vi "filter.test.vi"(9 "reset":bool, 10 "debug":bool) -> ()   [LabVIEW 2022 SP3]
uses:
  <vilib>/Platform/TimedLoop/XDataNode/timing_clust.ctl
  <vilib>/Platform/TimedLoop/XDataNode/nitl_modes.ctl
  <vilib>/Platform/TimedLoop/XDataNode/wakeup.ctl
  ticker.slot.ctl
  arty/orderbook/orderbook.command.ctl
  arty/orderbook/orderbook.command.type.ctl
  <vilib>/rvi/DataTransferAndStorage/Container/Common/niFpgaContainerGetUniqueNameForEmu.vi
  <vilib>/rvi/DataTransferAndStorage/Container/Common/niFpgaContainerSetEmuInfo.vi
  <vilib>/rvi/eio/common/nirviEmuReportErrorAndStop.vi
  <vilib>/rvi/Emulation/niFpgaSctlEmulationGetInTimedLoop.vi
  <vilib>/rvi/Emulation/niFpgaEmulationReportErrorSimple.vi
  <vilib>/rvi/Emulation/niFpgaGetClockAttributes.vi
  <vilib>/rvi/Emulation/niFpgaCriticalErrorInLSC.vi
  <vilib>/rvi/DataTransferAndStorage/Container/Common/niFpgaContainerExecOnDevCompGetState.vi
  <vilib>/rvi/Emulation/niFpgaEmulationIsFPGAContextNoSignature.vi
  <vilib>/rvi/errors/niFpgaSetErrorForExecOnDevCompSimple.vi
  <vilib>/rvi/FIFO/Fifo_Resource/nirvififoEmulationSetSize.vi
  <vilib>/rvi/FIFO/Fifo_Resource/nirviFifoEmulationQueueMgr.vi
  <instcachedir>/0/nirviFifoEmulationQueueMgr_E5CAEC123FF24DC58D834DCA3CDAA9B5.lvgen/nirviFifoEmulationQueueMgr_E5CAEC123FF24DC58D834DCA3CDAA9B5_012.vi
  <vilib>/rvi/FIFO/Fifo_Resource/nirvififoEmulationDetermineInputValidOut.vi
  <vilib>/rvi/FIFO/Fifo_Resource/nirvififoEmulationCreateLock.vi
  <vilib>/rvi/Emulation/niFpgaProcessEmulError.vi
  <vilib>/rvi/FIFO/Fifo_Resource/nirvififoEmulationObtainLock.vi
  <vilib>/rvi/FIFO/Fifo_Resource/nirvififoEmulationReleaseLock.vi
  <vilib>/rvi/occurrence/nirviWaitOnOccurrenceBase.vi
  <vilib>/rvi/errors/nirviReportUnexpectedCaseInternalError.vi
  <vilib>/rvi/errors/nirviReportUnexpectedCaseInternalError (U32).vi
  <vilib>/Utility/error.llb/Clear Errors.vi
  <vilib>/rvi/interface/RandomDataEmulation/niFpgaRandomDataHandleErrors.vi
  <instcachedir>/0/nirviFifoEmulationQueueMgr_E5CAEC123FF24DC58D834DCA3CDAA9B5.lvgen/nirviFifoEmulationQueueMgr_E5CAEC123FF24DC58D834DCA3CDAA9B5_011.vi
  <vilib>/rvi/interface/RandomDataEmulation/nirviRandomDataMultiElementFPGAFIFO.vi
  <instcachedir>/0/nirviRandomDataMultiElementFPGAFIFO_3E9965BA1FAD4E7B8DABA31768A09B1F.lvgen/nirviRandomDataMultiElementFPGAFIFO_3E9965BA1FAD4E7B8DABA31768A09B1F_001.vi
  <instcachedir>/0/nirviFifoEmulationQueueMgr_E5CAEC123FF24DC58D834DCA3CDAA9B5.lvgen/nirviFifoEmulationQueueMgr_E5CAEC123FF24DC58D834DCA3CDAA9B5_017.vi
  <vilib>/Platform/TimedLoop/XDataNode/XDataNode.xnode
  <vilib>/rvi/LocalResourceManager/LocalResourceManager.xnode
  <vilib>/rvi/DataTransferAndStorage/Container/XNode/niFpgaContainer.xnode
  <vilib>/rvi/FIFO/Fifo_Resource/niFpgaFifoEmulationRefIn.vi
  <vilib>/rvi/interface/RandomDataEmulation/nirviRandomDataFpgaReadWriteTemplate.vi
  <vilib>/rvi/FIFO/Fifo_Resource/nirvififoEmulationRead.vi
  <vilib>/rvi/interface/RandomDataEmulation/nirviRandomDataFpgaMultiElementTemplate.vi
  <vilib>/rvi/FIFO/Fifo_Resource/nirvififoEmulationWrite.vi
  <vilib>/Platform/TimedLoop/XDataNode/XDNodeRunTimeDep.lvlib
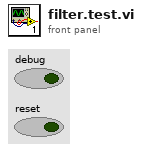
[diagram p1: front panel]
types:
  T1 = typedef "XDNodeRunTimeDep.lvlib/timing_clust.ctl" = cluster{"Expected End [f-1]":u64, "Actual End [f-1]":u64, "Finished Late? [f-1]":bool, "Expected End [i-1]":u64, "Actual End [i-1]":u64, "Finished Late? [i-1]":bool, "Expected Start [i]":u64, "Actual Start [i]":u64, "Expected Start [f]":u64, "Actual Start [f]":u64, "Source Name":string, "Structure Name":string, "Period":i64, "Deadline":i64, "Offset":i64, "Start":i64, "Priority":i32, "Timeout":i32, "Mode":T2, "Wakeup Reason":T3, "Error":errorcluster, "Source Type":string, "Secondary Source Type":string, "Global End Time":u64, "Global Start Time":u64, "Frame Duration":u64, "Iteration Duration":u64, "Assigned CPU":i32, "I/O Scan Engine Mode":u32}
  T2 = typedef "XDNodeRunTimeDep.lvlib/nitl_modes.ctl" = enum32{"No Change", "Process missed periods, maintain original phase", "Discard missed periods, maintain original phase", "Process missed periods, ignore original phase", "Discard missed periods, ignore original phase"}
  T3 = typedef "XDNodeRunTimeDep.lvlib/wakeup.ctl" = enum32{"Normal", "Aborted", "Asynchronous wakeup", "Timing source error", "Timed loop error", "Timeout"}
  T4 = typedef "orderbook.command.ctl" = cluster{"OrderBook Command.Type":T5, "Side (U8)":u8, "Order Id (U64)":u64, "Quantity (U32)":u32, "Symbol (U64)":u64, "Price (U64)":u64, "Executed Quantity (U32)":u32, "Canceled Quantity (U32)":u32, "Remaining Quantity (U32)":u32, "Seconds (U64)":u64, "Nanoseconds (U64)":u64}
  T5 = typedef "orderbook.command.type.ctl" = enum16{"Time", "AddOrder", "OrderExecuted", "OrderExecutedAtPrice", "ReduceSize", "ModifyOrder", "DeleteOrder", "Get.All.Orders", "Get.Top"}
  T6 = typedef "ticker.slot.ctl" = cluster{"Symbol":u64}
  T7 = cluster{"OrderBook Command.Type":enum16{"Time", "AddOrder", "OrderExecuted", "OrderExecutedAtPrice", "ReduceSize", "ModifyOrder", "DeleteOrder", "Get.All.Orders", "Get.Top"}, "Side (U8)":u8, "Order Id (U64)":u64, "Quantity (U32)":u32, "Symbol (U64)":u64, "Price (U64)":u64, "Executed Quantity (U32)":u32, "Canceled Quantity (U32)":u32, "Remaining Quantity (U32)":u32, "Seconds (U64)":u64, "Nanoseconds (U64)":u64}
  T8 = enum16{"Time", "AddOrder", "OrderExecuted", "OrderExecutedAtPrice", "ReduceSize", "ModifyOrder", "DeleteOrder", "Get.All.Orders", "Get.Top"}
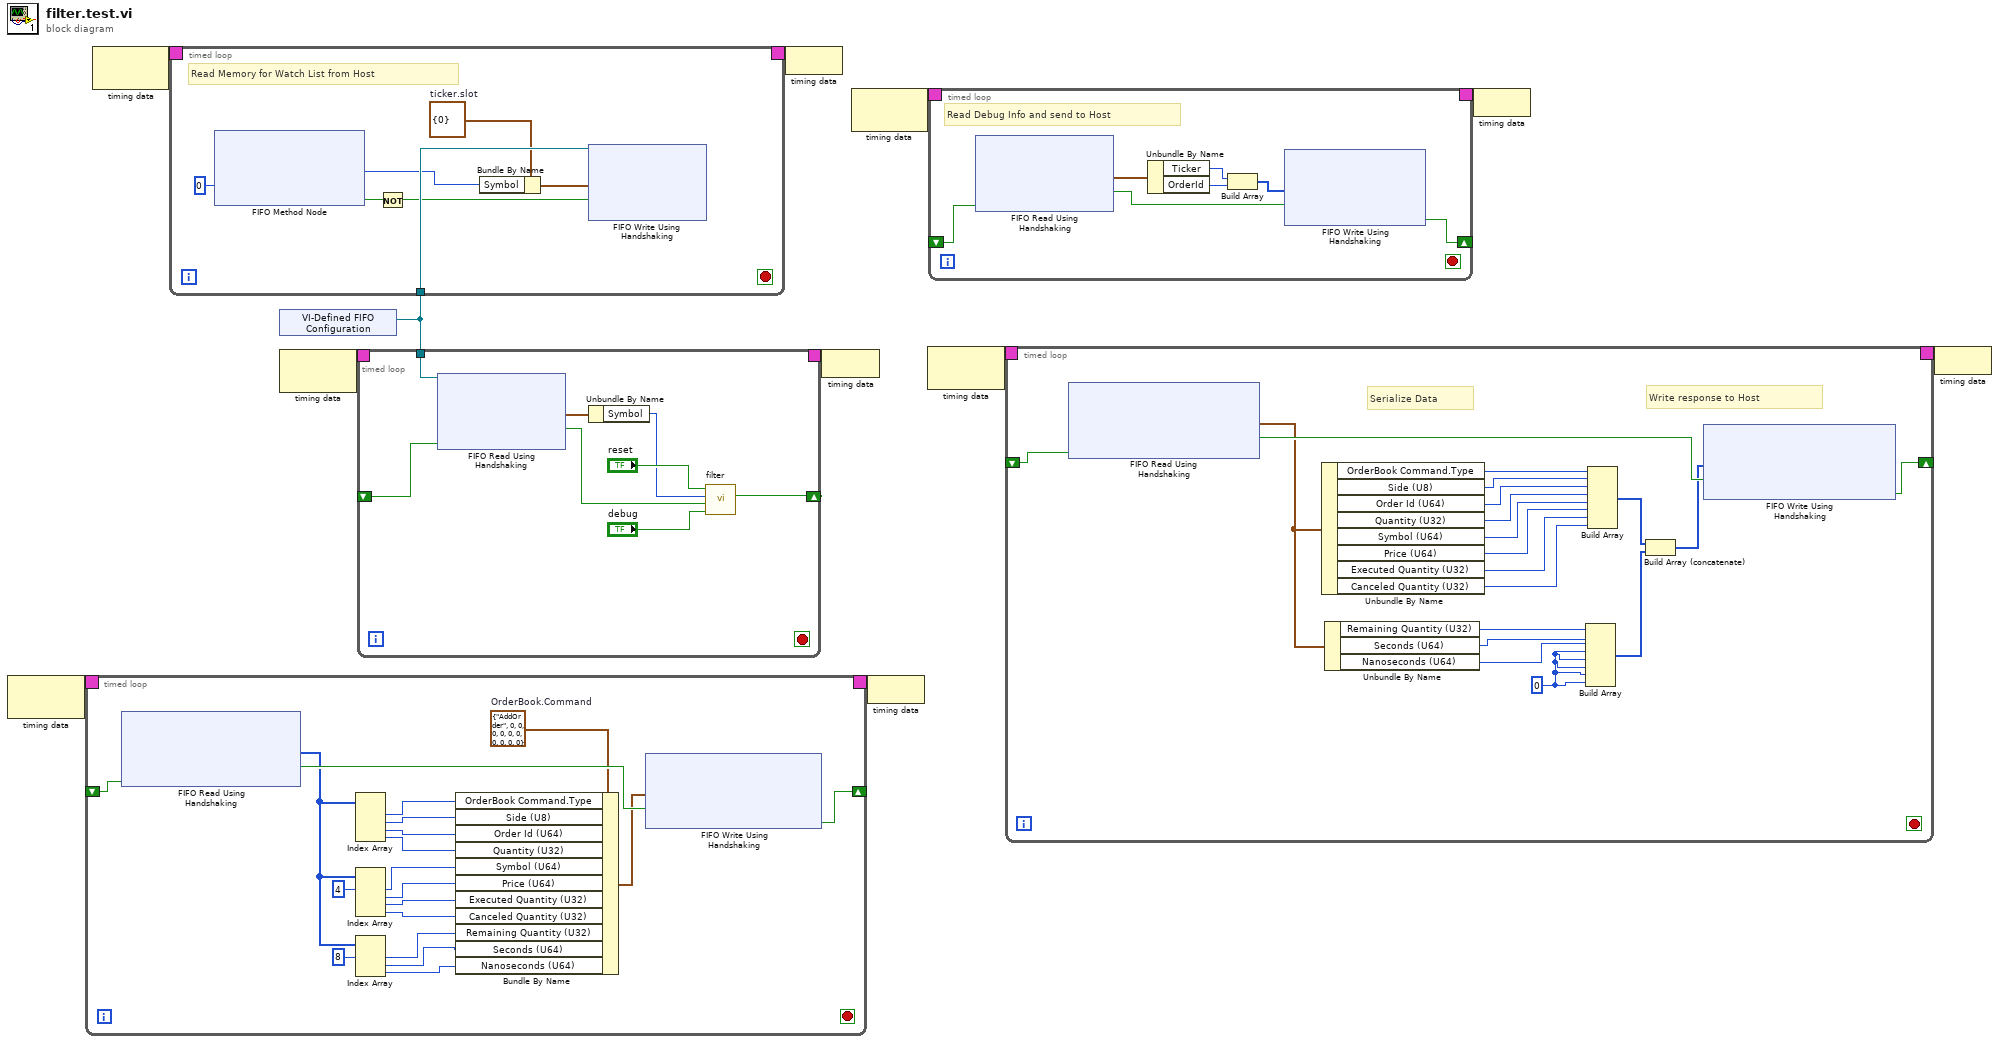
[diagram p0: block diagram]
diagram:
  n1 = node-c288() -> (w4:T1)  [unwired: 1 in]
  n2 = timed-loop {
    timing: w4 -> [_]
    timing-out: [_] -> w3
    shift-right: [w30] -> _
    shift-left: _ -> [w29]
    stop <- _ stop-if-true
    w27 = T4 {"OrderBook Command.Type"=enum."AddOrder", "Side (U8)"=0, "Order Id (U64)"=0, "Quantity (U32)"=0, "Symbol (U64)"=0, "Price (U64)"=0, "Executed Quantity (U32)"=0, "Canceled Quantity (U32)"=0, "Remaining Quantity (U32)"=0, "Seconds (U64)"=0, "Nanoseconds (U64)"=0}  # OrderBook.Command
    n3 = xnode ("FIFO Read Using Handshaking")("Ready for Output"=w29) -> ("Element"=w25:u64[], "Output Valid"=w28:bool)  [unwired: 1 in, 1 out]
    n4 = Index Array(array=w25) -> (element #1=w22:u64, element #2=w21:u64, element #3=w20:u64, element #4=w19:u64)  [unwired: 4 in]
    n5 = Index Array(array=w25, index #1=4 ("index")) -> (element #1=w18:u64, element #2=w17:u64, element #3=w16:u64, element #4=w15:u64)  [unwired: 3 in]
    n6 = Index Array(array=w25, index #1=8 ("index")) -> (element #1=w14:u64, element #2=w13:u64, element #3=w12:u64)  [unwired: 2 in]
    n7 = Bundle By Name(cluster=w27, "OrderBook Command.Type"=w22, "Side (U8)"=w21, "Order Id (U64)"=w20, "Quantity (U32)"=w19, "Symbol (U64)"=w18, "Price (U64)"=w17, "Executed Quantity (U32)"=w16, "Canceled Quantity (U32)"=w15, "Remaining Quantity (U32)"=w14, "Seconds (U64)"=w13, "Nanoseconds (U64)"=w12) -> (w26:T4)
    n8 = xnode ("FIFO Write Using Handshaking")("Element"=w26, "Input Valid"=w28) -> ("Ready for Input"=w30:bool)  [unwired: 1 in, 1 out]
  }
  n9 = node-c288() -> (w9:T1)  [unwired: 1 in]
  n10 = xnode "VI-Defined FIFO Configuration"() -> ("FIFO Out"=w7:refnum<k21>)
  n11 = timed-loop {
    timing: w9 -> [_]
    timing-out: [_] -> w8
    tunnel: w7 -> [w38]
    stop <- _ stop-if-true
    w35 = T6 {"Symbol"=0}  # ticker.slot
    # "Read Memory for Watch List from Host"
    n12 = xnode ("FIFO Method Node")("Timeout"=0) -> ("Element"=w33:u64, "Timed Out?"=w37:bool)  [unwired: 1 in, 1 out]
    n13 = Not(x=w37) -> (.not. x?=w36:bool)
    n14 = Bundle By Name(cluster=w35, "Symbol"=w33) -> (w34:T6)
    n15 = xnode ("FIFO Write Using Handshaking")("Element"=w34, "Input Valid"=w36, "FIFO In"=w38) -> ()  [unwired: 2 out]
  }
  n16 = node-c288() -> (w11:T1)  [unwired: 1 in]
  n17 = timed-loop {
    timing: w11 -> [_]
    timing-out: [_] -> w10
    tunnel: w7 -> [w49]
    shift-right: [w44] -> _
    shift-left: _ -> [w43]
    stop <- _ stop-if-true
    n18 = xnode ("FIFO Read Using Handshaking")("Ready for Output"=w43, "FIFO In"=w49) -> ("Element"=w48:cluster{"Symbol":u64}, "Output Valid"=w46:bool)  [unwired: 1 out]
    n19 = Unbundle By Name(w48) -> ("Symbol"=w42:u64)
    n20 = call "filter.vi"("debug"="debug", "conf.valid"=w46, "conf"=w42, "reset"="reset") -> ("Ready.for.Configuration.Input"=w44:bool)  [unwired: 6 in, 1 out]
  }
  n21 = node-c288(w8) -> ()
  n22 = node-c288(w10) -> ()
  n23 = node-c288() -> (w6:T1)  [unwired: 1 in]
  n24 = node-c288(w3) -> ()
  n25 = node-c288() -> (w2:T1)  [unwired: 1 in]
  n26 = timed-loop {
    timing: w6 -> [_]
    timing-out: [_] -> w5
    shift-right: [w58] -> _
    shift-left: _ -> [w57]
    stop <- _ stop-if-true
    # "Read Debug Info and send to Host"
    n27 = xnode ("FIFO Read Using Handshaking")("Ready for Output"=w57) -> ("Element"=w55:cluster{"Ticker":u64, "OrderId":u64}, "Output Valid"=w56:bool)  [unwired: 1 in, 1 out]
    n28 = Unbundle By Name(w55) -> ("Ticker"=w53:u64, "OrderId"=w54:u64)
    n29 = Build Array(w53, w54) -> (w52:u64[])
    n30 = xnode ("FIFO Write Using Handshaking")("Element"=w52, "Input Valid"=w56) -> ("Ready for Input"=w58:bool)  [unwired: 1 in, 1 out]
  }
  n31 = timed-loop {
    timing: w2 -> [_]
    timing-out: [_] -> w1
    shift-right: [w79] -> _
    shift-left: _ -> [w70]
    stop <- _ stop-if-true
    w63 = u64 0 ("element")
    # "Serialize Data"
    # "Write response to Host"
    n32 = xnode ("FIFO Read Using Handshaking")("Ready for Output"=w70) -> ("Element"=w65:T7, "Output Valid"=w69:bool)  [unwired: 1 in, 1 out]
    n33 = Unbundle By Name(w65) -> ("OrderBook Command.Type"=w78:T8, "Side (U8)"=w77:u8, "Order Id (U64)"=w76:u64, "Quantity (U32)"=w75:u32, "Symbol (U64)"=w74:u64, "Price (U64)"=w73:u64, "Executed Quantity (U32)"=w72:u32, "Canceled Quantity (U32)"=w71:u32)
    n34 = Unbundle By Name(w65) -> ("Remaining Quantity (U32)"=w64:u32, "Seconds (U64)"=w61:u64, "Nanoseconds (U64)"=w62:u64)
    n35 = Build Array(w64, w61, w62, w63, w63, w63, w63, w63) -> (w66:u64[])
    n36 = Build Array(w78, w77, w76, w75, w74, w73, w72, w71) -> (w68:u64[])
    n37 = Build Array (concatenate)(w68, w66) -> (w67:u64[])
    n38 = xnode ("FIFO Write Using Handshaking")("Element"=w67, "Input Valid"=w69) -> ("Ready for Input"=w79:bool)  [unwired: 1 in, 1 out]
  }
  n39 = node-c288(w5) -> ()
  n40 = node-c288(w1) -> ()
